vi "tlc_controller_main.vi"(7 "Command (Check State)":T1=enum."Check State", 8 "error in (no error)":errorcluster, 11 "Sensors":T5) -> (0 "error out":errorcluster, 3 "Traffic Lights":T2)   [LabVIEW 2009]
doc: "This VI is the Main VI for the Controller module. This module is responsible for controlling the states of the Traffic Lights and from moving from one state to the next based on the Sensors input and previous state information. The module will output the Traffic Lights that can be used to update the display in the UI.\n\nThe states, transition logic and the time in which the controller stays in the state are as follows:\nN/S Green (4s)\nN/S Yellow (2s)\nAll Red (2s)\nIf East Sensor OR West Sensor = TRUE then\n E/W Left Green (4s)\n E/W Left Yellow (2s)\n All Red (2s)\nE/W Green (4s)\nE/W Yellow (2s)\nAll Red (2s)\nIf North Sensor or South Sensor = TRUE then\n N/s Left Green (4s)\n N/S Left Yellow (2s)\n All Red (2s)\n<repeat>\n\nSee the Block Diagram for more detailed information."
uses:
  tlc_controller_SensorData_cluster.ctl
  tlc_controller_TrafficLightsData_cluster.ctl
  controls/tlc_TrafficLightDisplay_cluster.ctl
  controls/tlc_TrafficLightLeftDisplay_cluster.ctl
  tlc_controller_Command_enum.ctl
  timer/tlc_timer_Command_enum.ctl
  tlc_controller_StateTimes_cluster.ctl
  tlc_controller_TrafficLightState_enum.ctl
panel:
  # "Inputs"
  # "Outputs"
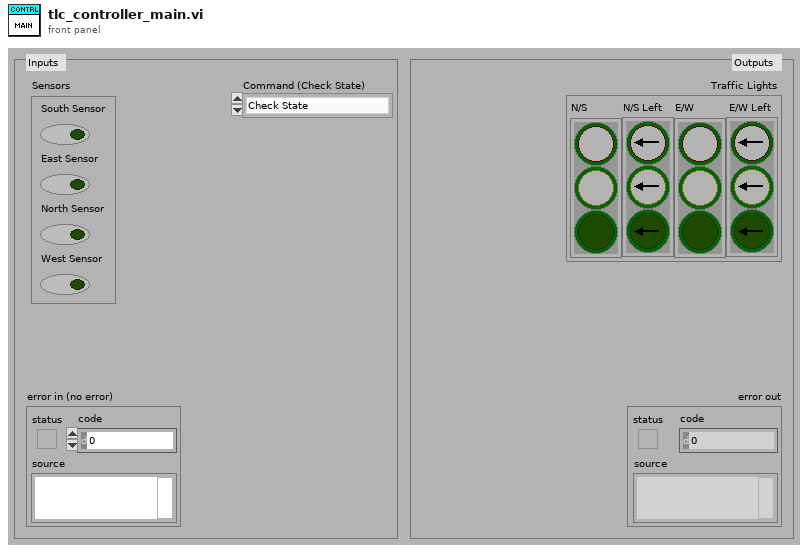
[diagram p1: front panel]
types:
  T1 = typedef "tlc_controller_Command_enum.ctl" = enum16{"Initialise", "Check State", "Next State Logic", "Set Traffic Lights", "Shutdown"}
  T2 = typedef "tlc_controller_TrafficLightsData_cluster.ctl" = cluster{"N/S":T3, "N/S Left":T4, "E/W":T3, "E/W Left":T4}
  T3 = typedef "tlc_TrafficLightDisplay_cluster.ctl" = cluster{"Red":bool, "Yellow":bool, "Green":bool}
  T4 = typedef "tlc_TrafficLightLeftDisplay_cluster.ctl" = cluster{"Red":bool, "Yellow":bool, "Green":bool}
  T5 = typedef "tlc_controller_SensorData_cluster.ctl" = cluster{"South Sensor":bool, "East Sensor":bool, "North Sensor":bool, "West Sensor":bool}
  T6 = typedef "tlc_timer_Command_enum.ctl" = enum16{"Start Timer", "Check Timer"}
  T7 = typedef "tlc_controller_TrafficLightState_enum.ctl" = enum16{"All Red", "N/S Green", "N/S Yellow", "E/W Left Green", "E/W Left Yellow", "E/W Green", "E/W Yellow", "N/S Left Green", "N/S Left Yellow"}
  T8 = typedef "tlc_controller_StateTimes_cluster.ctl" = cluster{"Green":dbl, "Yellow":dbl, "Red":dbl}
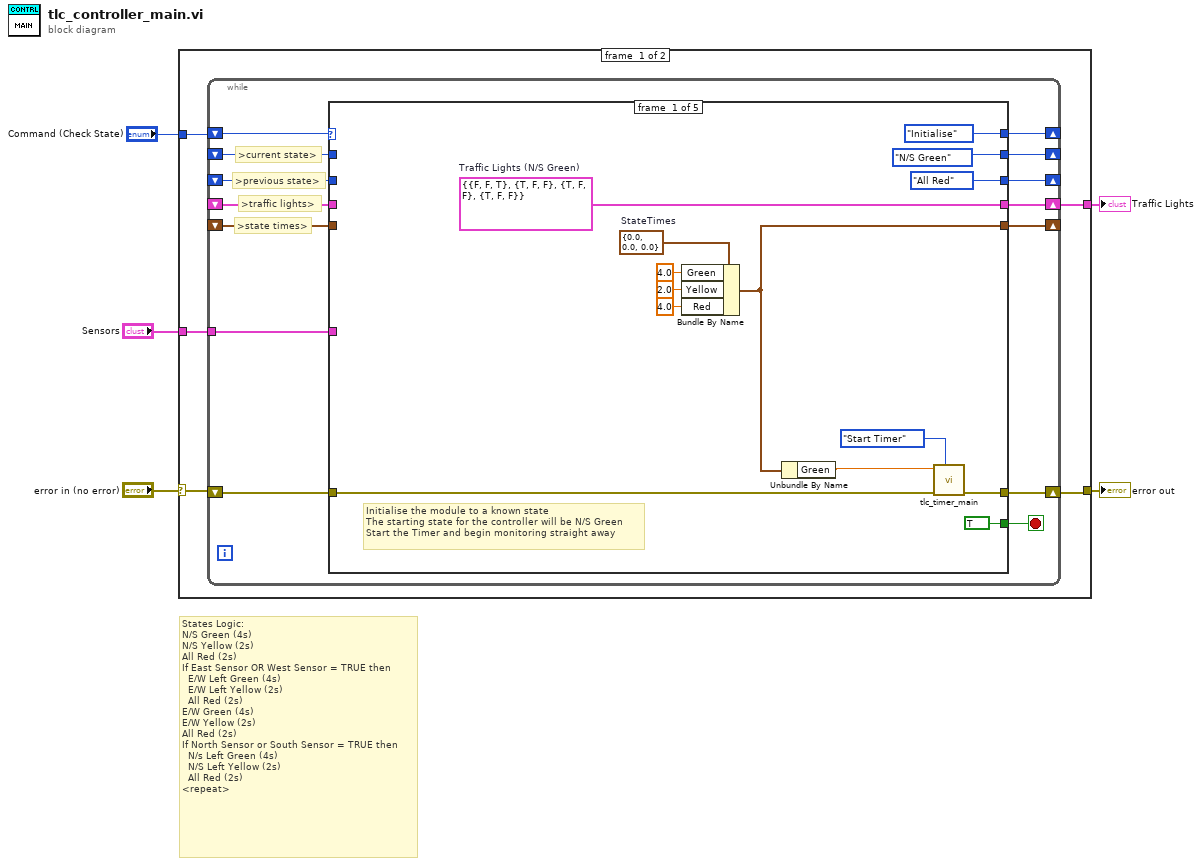
[diagram p0: block diagram]
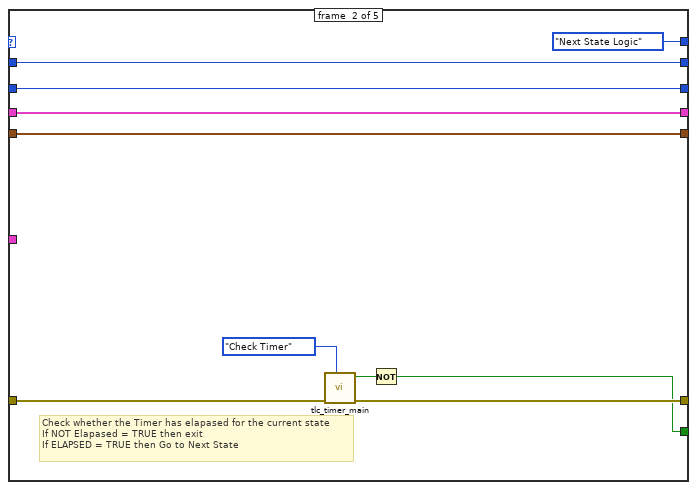
[diagram p2: hidden frame]
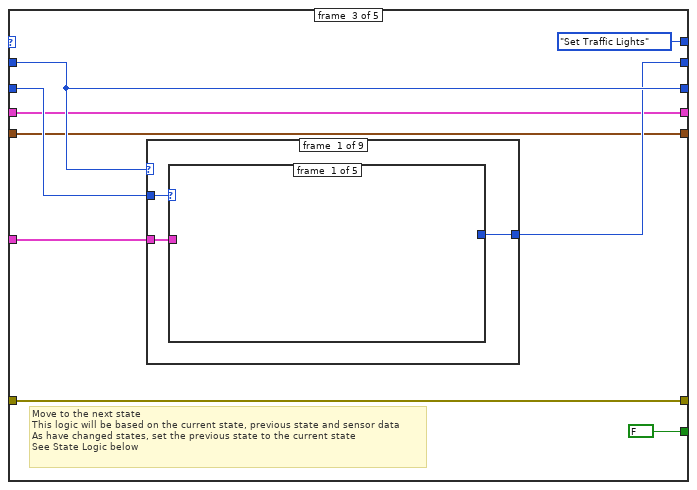
[diagram p3: hidden frame]
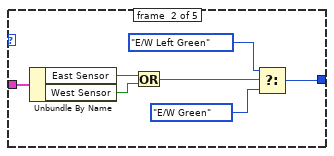
[diagram p4: hidden frame]
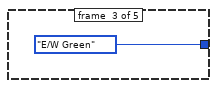
[diagram p5: hidden frame]
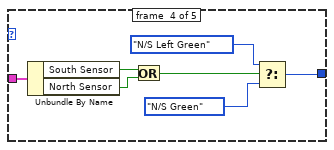
[diagram p6: hidden frame]
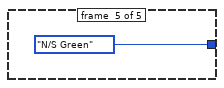
[diagram p7: hidden frame]
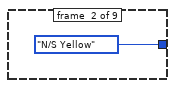
[diagram p8: hidden frame]
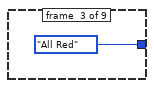
[diagram p9: hidden frame]
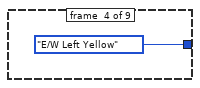
[diagram p10: hidden frame]
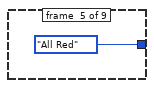
[diagram p11: hidden frame]
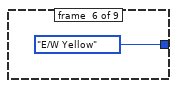
[diagram p12: hidden frame]
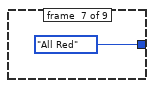
[diagram p13: hidden frame]
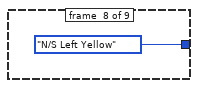
[diagram p14: hidden frame]
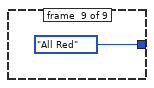
[diagram p15: hidden frame]
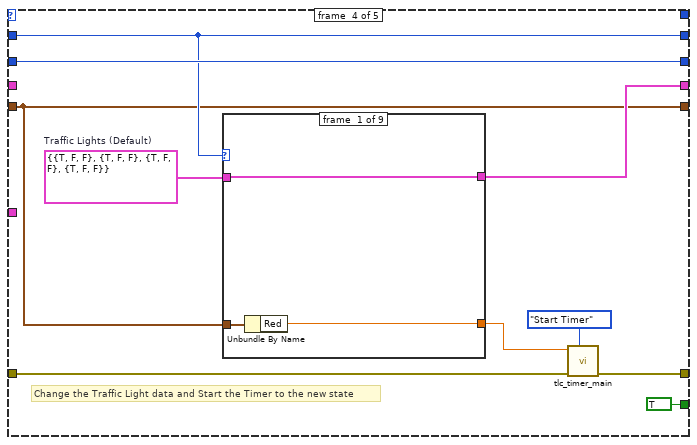
[diagram p16: hidden frame]
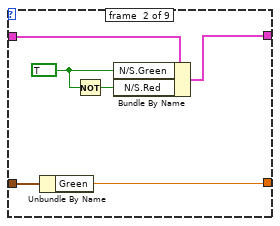
[diagram p17: hidden frame]
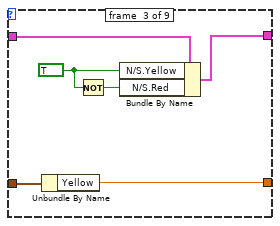
[diagram p18: hidden frame]
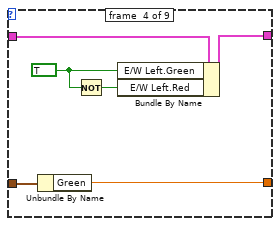
[diagram p19: hidden frame]
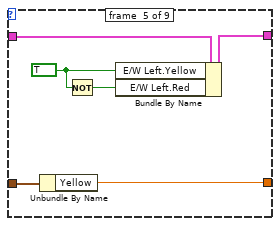
[diagram p20: hidden frame]
diagram:
  # "States Logic:\nN/S Green (4s)\nN/S Yellow (2s)\nAll Red (2s)\nIf East Sensor OR West Sensor = TRUE then\n  E/W Left Green (4s)\n  E/W Left Yellow (2s)\n  All Red (2s)\nE/W Green (4s)\nE/W Yellow (2s)\nAll Red (2s)\nIf North Sensor or South Sensor = TRUE then\n  N/s Left Green (4s)\n  N/S Left Yellow (2s)\n  All Red (2s)\n<repeat>"
  n1 = case shown="No Error" "error in (no error)" {
    selector: "error in (no error)" -> [w10 w152]
    tunnel: [w9 w152] -> w4
    tunnel: "Sensors" -> [w8 _]
    tunnel: "Command (Check State)" -> [w6 _]
    tunnel: [w7 _] -> w1
    frame #0 {
      n2 = while {
        shift-right: [w24] -> w9
        shift-left: w10 -> [w23]
        shift-right: [w19] -> _
        shift-left: _ -> [w21]
        shift-right: [w18] -> _
        shift-left: _ -> [w20]
        tunnel: w8 -> [w17]
        shift-right: [w15] -> w7
        shift-left: _ -> [w16]
        shift-right: [w13] -> _
        shift-left: w6 -> [w14]
        shift-right: [w12] -> _
        shift-left: _ -> [w11]
        stop <- w22 stop-if-true
        # ">state times>"
        # ">traffic lights>"
        # ">previous state>"
        # ">current state>"
        n3 = case shown="\"Set Traffic Lights\"" w14 {
          tunnel: [w27 w43 w50 w86 w151] -> w24
          tunnel: w23 -> [w28 w44 w50 w87 w151]
          tunnel: [TRUE w41 FALSE TRUE TRUE] -> w22
          tunnel: w21 -> [_ w48 w56 w93 w147]
          tunnel: w20 -> [_ w47 w55 w94 w148]
          tunnel: [tlc_controller_TrafficLightState_enum."N/S Green" ("Traffic Light State") w48 w53 w93 w147] -> w19
          tunnel: [tlc_controller_TrafficLightState_enum."All Red" ("Traffic Light State") w47 w56 w94 w148] -> w18
          tunnel: w17 -> [_ _ w54 _ _]
          tunnel: w16 -> [_ w46 w52 _ w149]
          tunnel: [w36 w46 w52 w91 w149] -> w15
          tunnel: [tlc_controller_Command_enum."Initialise" ("Command (Check State)") tlc_controller_Command_enum."Next State Logic" ("Command (Check State)") tlc_controller_Command_enum."Set Traffic Lights" ("Command (Check State)") _ _] -> w13
          tunnel: [w26 w39 w49 w89 w146] -> w12
          tunnel: w11 -> [_ w39 w49 w89 w146]
          frame #0 {
            w33 = T8 {"Green"=0.0, "Yellow"=0.0, "Red"=0.0}  # StateTimes
            w36 = T2 {"N/S"={"Red"=FALSE, "Yellow"=FALSE, "Green"=TRUE}, "N/S Left"={"Red"=TRUE, "Yellow"=FALSE, "Green"=FALSE}, "E/W"={"Red"=TRUE, "Yellow"=FALSE, "Green"=FALSE}, "E/W Left"={"Red"=TRUE, "Yellow"=FALSE, "Green"=FALSE}}  # Traffic Lights (N/S Green)
            # "Initialise the module to a known state\nThe starting state for the controller will be N/S Green\nStart the Timer and begin monitoring straight away"
            n4 = Bundle By Name(cluster=w33, "Green"=4.0, "Yellow"=2.0, "Red"=4.0) -> (w26:T8)
            n5 = Unbundle By Name(w26) -> ("Green"=w25:dbl)
            n6 = call "tlc_timer_main.vi"("Command (Check Timer)"=tlc_timer_Command_enum."Start Timer", "error in (no error)"=w28, "Target Time (s)"=w25) -> ("error out"=w27:errorcluster)  [unwired: 7 in, 1 out]
          }
          frame #1 {
            # "Check whether the Timer has elapased for the current state\nIf NOT Elapased = TRUE then exit\nIf ELAPSED = TRUE then Go to Next State"
            n7 = call "tlc_timer_main.vi"("Command (Check Timer)"=tlc_timer_Command_enum."Check Timer", "error in (no error)"=w44) -> ("error out"=w43:errorcluster, "Elapsed"=w42:bool)  [unwired: 8 in]
            n8 = Not(x=w42) -> (.not. x?=w41:bool)
          }
          frame #2 {
            # "Move to the next state\nThis logic will be based on the current state, previous state and sensor data\nAs have changed states, set the previous state to the current state \nSee State Logic below"
            n9 = case shown="\"All Red\"" w56 {
              tunnel: w55 -> [w60 _ _ _ _ _ _ _ _]
              tunnel: w54 -> [w59 _ _ _ _ _ _ _ _]
              tunnel: [w58 tlc_controller_TrafficLightState_enum."N/S Yellow" ("Traffic Light State") tlc_controller_TrafficLightState_enum."All Red" ("Traffic Light State") tlc_controller_TrafficLightState_enum."E/W Left Yellow" ("Traffic Light State") tlc_controller_TrafficLightState_enum."All Red" ("Traffic Light State") tlc_controller_TrafficLightState_enum."E/W Yellow" ("Traffic Light State") tlc_controller_TrafficLightState_enum."All Red" ("Traffic Light State") tlc_controller_TrafficLightState_enum."N/S Left Yellow" ("Traffic Light State") tlc_controller_TrafficLightState_enum."All Red" ("Traffic Light State")] -> w53
              frame #0 {
                n10 = case shown="\"E/W Left Yellow\"" w60 {
                  tunnel: w59 -> [_ w67 _ w75 _]
                  tunnel: [_ w61 tlc_controller_TrafficLightState_enum."E/W Green" ("Traffic Light State") w69 tlc_controller_TrafficLightState_enum."N/S Green" ("Traffic Light State")] -> w58
                  frame #0 {
                  }
                  frame #1 {
                    n11 = Unbundle By Name(w67) -> ("East Sensor"=w66:bool, "West Sensor"=w65:bool)
                    n12 = Or(x=w66, y=w65) -> (x .or. y?=w64:bool)
                    n13 = Select(t=tlc_controller_TrafficLightState_enum."E/W Left Green" ("Traffic Light State"), s=w64, f=tlc_controller_TrafficLightState_enum."E/W Green" ("Traffic Light State")) -> (s? t:f=w61:T7)
                  }
                  frame #2 {
                  }
                  frame #3 {
                    n14 = Unbundle By Name(w75) -> ("South Sensor"=w74:bool, "North Sensor"=w73:bool)
                    n15 = Or(x=w74, y=w73) -> (x .or. y?=w72:bool)
                    n16 = Select(t=tlc_controller_TrafficLightState_enum."N/S Left Green" ("Traffic Light State"), s=w72, f=tlc_controller_TrafficLightState_enum."N/S Green" ("Traffic Light State")) -> (s? t:f=w69:T7)
                  }
                  frame #4 {
                  }
                }
              }
              frame #1 {
              }
              frame #2 {
              }
              frame #3 {
              }
              frame #4 {
              }
              frame #5 {
              }
              frame #6 {
              }
              frame #7 {
              }
              frame #8 {
              }
            }
          }
          frame #3 {
            w92 = T2 {"N/S"={"Red"=TRUE, "Yellow"=FALSE, "Green"=FALSE}, "N/S Left"={"Red"=TRUE, "Yellow"=FALSE, "Green"=FALSE}, "E/W"={"Red"=TRUE, "Yellow"=FALSE, "Green"=FALSE}, "E/W Left"={"Red"=TRUE, "Yellow"=FALSE, "Green"=FALSE}}  # Traffic Lights (Default)
            # "Change the Traffic Light data and Start the Timer to the new state"
            n17 = case shown="\"All Red\"" w93 {
              tunnel: w92 -> [w95 w103 w109 w115 w121 w127 w133 w139 w145]
              tunnel: [w95 w102 w108 w114 w120 w126 w132 w138 w144] -> w91
              tunnel: w89 -> [w97 w101 w107 w113 w119 w125 w131 w137 w143]
              tunnel: [w96 w100 w106 w112 w118 w124 w130 w136 w142] -> w85
              frame #0 {
                n18 = Unbundle By Name(w97) -> ("Red"=w96:dbl)
              }
              frame #1 {
                w99 = TRUE ("N/S.Green")
                n19 = Unbundle By Name(w101) -> ("Green"=w100:dbl)
                n20 = Not(x=w99) -> (.not. x?=w98:bool)
                n21 = Bundle By Name(cluster=w103, "N/S.Green"=w99, "N/S.Red"=w98) -> (w102:T2)
              }
              frame #2 {
                w105 = TRUE ("N/S.Green")
                n22 = Unbundle By Name(w107) -> ("Yellow"=w106:dbl)
                n23 = Not(x=w105) -> (.not. x?=w104:bool)
                n24 = Bundle By Name(cluster=w109, "N/S.Yellow"=w105, "N/S.Red"=w104) -> (w108:T2)
              }
              frame #3 {
                w111 = TRUE ("N/S.Green")
                n25 = Unbundle By Name(w113) -> ("Green"=w112:dbl)
                n26 = Not(x=w111) -> (.not. x?=w110:bool)
                n27 = Bundle By Name(cluster=w115, "E/W Left.Green"=w111, "E/W Left.Red"=w110) -> (w114:T2)
              }
              frame #4 {
                w117 = TRUE ("N/S.Green")
                n28 = Unbundle By Name(w119) -> ("Yellow"=w118:dbl)
                n29 = Not(x=w117) -> (.not. x?=w116:bool)
                n30 = Bundle By Name(cluster=w121, "E/W Left.Yellow"=w117, "E/W Left.Red"=w116) -> (w120:T2)
              }
              frame #5 {
                w123 = TRUE ("N/S.Green")
                n31 = Unbundle By Name(w125) -> ("Green"=w124:dbl)
                n32 = Not(x=w123) -> (.not. x?=w122:bool)
                n33 = Bundle By Name(cluster=w127, "E/W.Green"=w123, "E/W.Red"=w122) -> (w126:T2)
              }
              frame #6 {
                w129 = TRUE ("N/S.Green")
                n34 = Unbundle By Name(w131) -> ("Yellow"=w130:dbl)
                n35 = Not(x=w129) -> (.not. x?=w128:bool)
                n36 = Bundle By Name(cluster=w133, "E/W.Yellow"=w129, "E/W.Red"=w128) -> (w132:T2)
              }
              frame #7 {
                w135 = TRUE ("N/S.Green")
                n37 = Unbundle By Name(w137) -> ("Green"=w136:dbl)
                n38 = Not(x=w135) -> (.not. x?=w134:bool)
                n39 = Bundle By Name(cluster=w139, "N/S Left.Green"=w135, "N/S Left.Red"=w134) -> (w138:T2)
              }
              frame #8 {
                w141 = TRUE ("N/S.Green")
                n40 = Unbundle By Name(w143) -> ("Yellow"=w142:dbl)
                n41 = Not(x=w141) -> (.not. x?=w140:bool)
                n42 = Bundle By Name(cluster=w145, "N/S Left.Yellow"=w141, "N/S Left.Red"=w140) -> (w144:T2)
              }
            }
            n43 = call "tlc_timer_main.vi"("Command (Check Timer)"=tlc_timer_Command_enum."Start Timer", "error in (no error)"=w87, "Target Time (s)"=w85) -> ("error out"=w86:errorcluster)  [unwired: 7 in, 1 out]
          }
          frame #4 {
            # "Run shutdown procedure (if required)"
          }
        }
      }
    }
    frame #1 {
    }
  }
  "error out" <- w4
  "Traffic Lights" <- w1
